vi "Init Controls.vi"(8 "error in (no error)":errorcluster, 11 "Editor in":refnum<class "Editor.lvclass">) -> (0 "error out":errorcluster, 3 "Editor out":refnum<class "Editor.lvclass">)   [LabVIEW 2020, in "VolatusGUIEditor.lvlib" / "Editor.lvclass"]
uses:
  Editor.lvclass
  Control List/Control List.lvclass
  Editor.lvclass/Editor.ctl
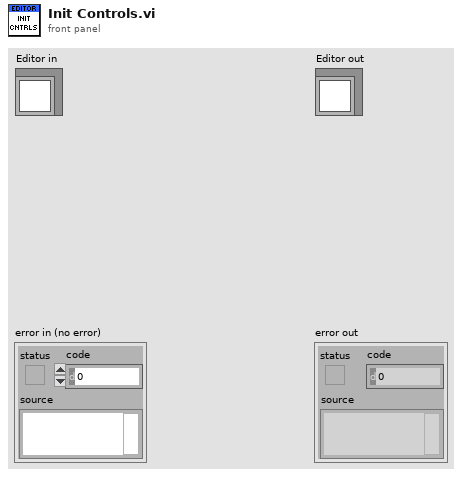
[diagram p1: front panel]
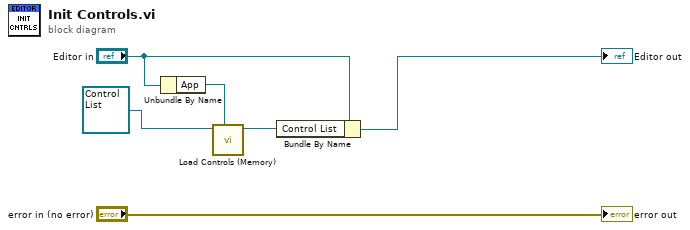
[diagram p0: block diagram]
diagram:
  n1 = Unbundle By Name("Editor in") -> ("App"=w2:refnum<vi>)
  n2 = call "Load Controls (Memory).vi"("App"=w2, "Control List in"=refnum<class "Control List.lvclass"> refnum ("VolatusGUIEditor.lvlib:Control List.lvclass")) -> ("Control List out"=w1:refnum<class "Control List.lvclass">)  [unwired: 8 in, 1 out]
  n3 = Bundle By Name(cluster="Editor in", "Control List"=w1) -> (→"Editor out":refnum<class "Editor.lvclass">)
  "error out" <- "error in (no error)"
